vi "S2C_M2p5942_Proc_ManageLoopError.vi"(8 "Error In":errorcluster) -> (0 "Error Out":errorcluster)   [LabVIEW 2024]
uses:
  S2C_M2p5942_Proc_Globals.vi
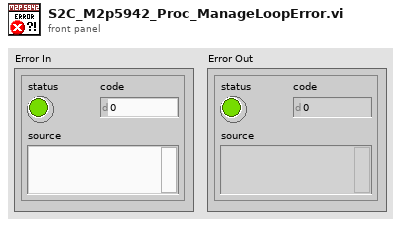
[diagram p1: front panel]
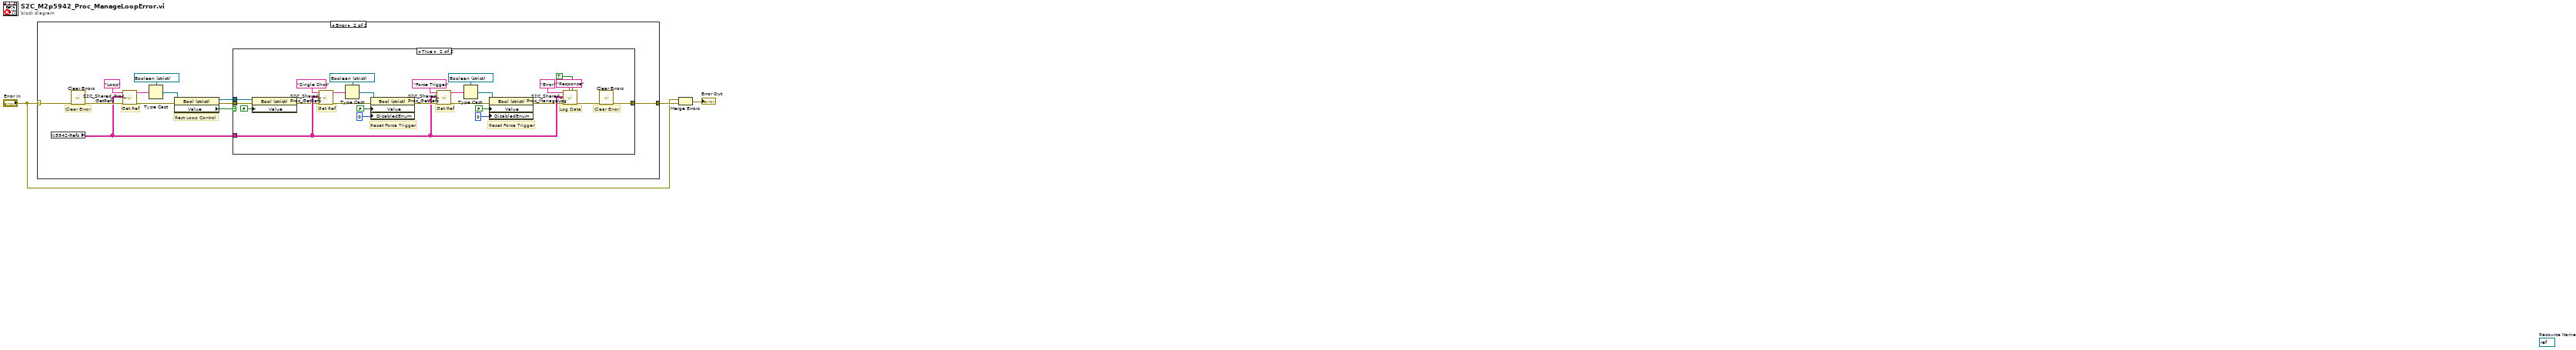
[diagram p0: block diagram]
diagram:
  (unwired) refnum<visa-resource-name> refnum  # Resource Name
  n1 = case shown="Error" "Error In" {
    selector: "Error In" -> [w4 w9]
    tunnel: [w4 w6] -> w3
    frame No Error {
    }
    frame Error {
      # "Rest Loop Control"
      # "Get Ref"
      # "Clear Error"
      n2 = global read "S2C_M2p5942_Proc_Globals.vi" "5942-Refs"() -> (w8:string[][])
      n3 = call <vilib>:"Clear Errors.vi"("error in (no error)"=w9) -> ("error out"=w10:errorcluster)  [unwired: 5 in, 1 out]
      n4 = call "S2C_Shared_Proc_GetRefs.vi"("Error In"=w10, "Refs"=w8, "Label"="Loop") -> ("Error Out"=w16:errorcluster, "Reference"=w14:string)  [unwired: 7 in]
      n5 = Type Cast(type=refnum<vi> refnum ("Force Trigger?"), x=w14) -> (*(type *) &x=w15:refnum<vi>)
      n6 = property class="Bool (strict)"(reference=w15, error in=w16) -> (reference out=w5:refnum<vi>, error out=w11:errorcluster, "Value"=w7:bool)
      n7 = case shown="True" w7 {
        tunnel: w11 -> [w17 w18]
        tunnel: w8 -> [_ w22]
        tunnel: [w17 w25] -> w6
        tunnel: w5 -> [_ w24]
        frame False {
        }
        frame True {
          # "Clear Error"
          # "Log Data"
          # "Reset Force Trigger"
          # "Get Ref"
          # "Reset Force Trigger"
          # "Get Ref"
          n8 = property class="Bool (strict)"(reference=w24, error in=w18, "Value"=FALSE) -> (error out=w21:errorcluster)  [unwired: 1 out]
          n9 = call "S2C_Shared_Proc_GetRefs.vi"("Error In"=w21, "Refs"=w22, "Label"="Single Shot") -> ("Error Out"=w43:errorcluster, "Reference"=w41:string)  [unwired: 7 in]
          n10 = Type Cast(type=refnum<vi> refnum ("Force Trigger?"), x=w41) -> (*(type *) &x=w42:refnum<vi>)
          n11 = property class="Bool (strict)"(reference=w42, error in=w43, "Value"=FALSE, "DisabledEnum"=u8 0) -> (error out=w29:errorcluster)  [unwired: 1 out]
          n12 = call "S2C_Shared_Proc_GetRefs.vi"("Error In"=w29, "Refs"=w22, "Label"="Force Trigger") -> ("Error Out"=w30:errorcluster, "Reference"=w32:string)  [unwired: 7 in]
          n13 = Type Cast(type=refnum<vi> refnum ("Force Trigger?"), x=w32) -> (*(type *) &x=w31:refnum<vi>)
          n14 = property class="Bool (strict)"(reference=w31, error in=w30, "Value"=FALSE, "DisabledEnum"=u8 0) -> (error out=w20:errorcluster)  [unwired: 1 out]
          n15 = call "S2C_Shared_Proc_ManageLog.vi"("Local?"=TRUE, "Command"="Response", "Error In"=w20, "Refs"=w22, "Data In"="Error") -> ("Error Out"=w26:errorcluster)  [unwired: 5 in, 1 out]
          n16 = call <vilib>:"Clear Errors.vi"("error in (no error)"=w26) -> ("error out"=w25:errorcluster)  [unwired: 5 in, 1 out]
        }
      }
    }
  }
  n17 = Merge Errors("Error In", w3) -> (→"Error Out":errorcluster)
